vi "verify expouse time.vi"(8 "error in (no error)":errorcluster, 11 "Simulated_CCD_Camera in":refnum<class "Sim_CCD.lvclass">) -> (0 "error out":errorcluster, 3 "Simulated_CCD_Camera out":refnum<class "Sim_CCD.lvclass">)   [LabVIEW 2018, in "Sim_CCD.lvclass"]
uses:
  Sim_CCD.lvclass
  Sim_CCD.lvclass/Sim_CCD.ctl
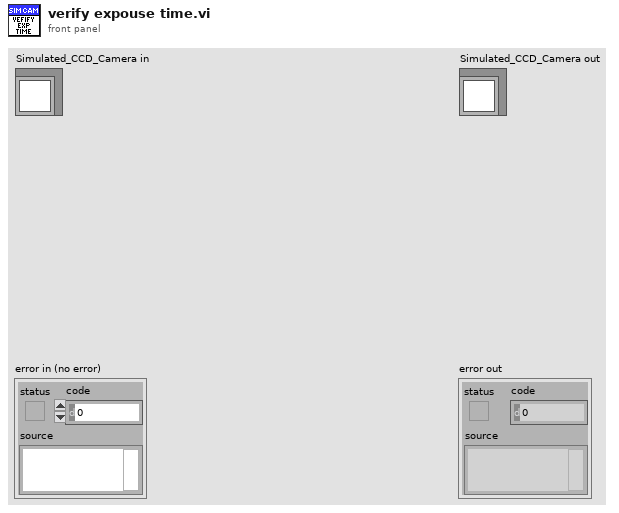
[diagram p1: front panel]
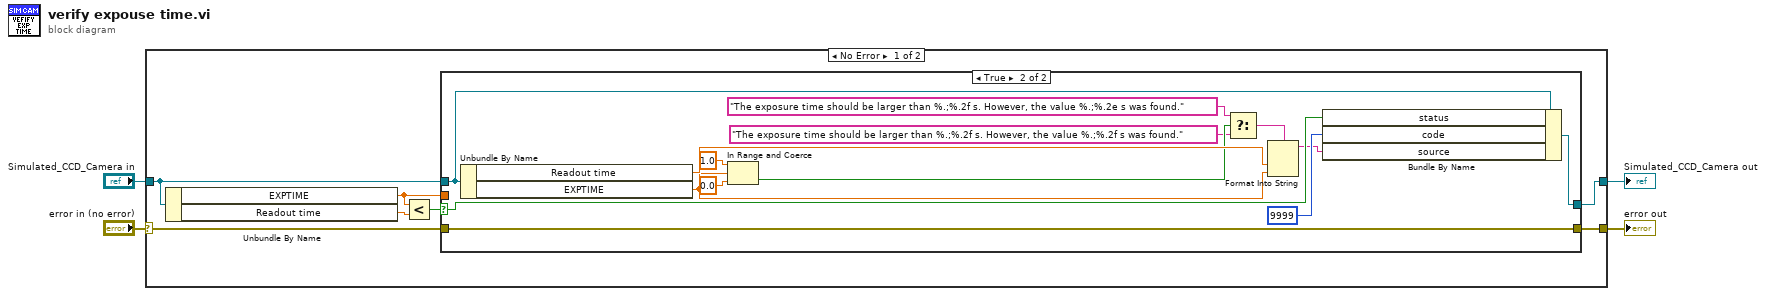
[diagram p0: block diagram]
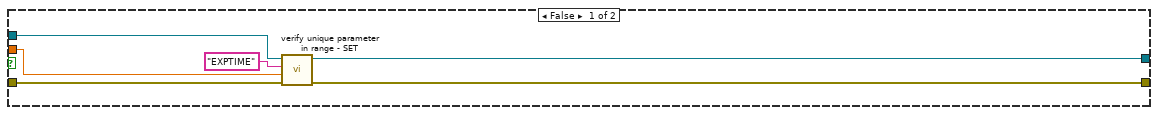
[diagram p2: hidden frame]
diagram:
  n1 = case shown="No Error" "error in (no error)" {
    selector: "error in (no error)" -> [w8 w33]
    tunnel: [w6 w33] -> w3
    tunnel: [w9 w32] -> w2
    tunnel: "Simulated_CCD_Camera in" -> [w5 w32]
    frame No Error {
      n2 = Unbundle By Name(w5) -> ("EXPTIME"=w7:dbl, "Readout time"=w11:dbl)
      n3 = Less?(x=w7, y=w11) -> (x < y?=w10:bool)
      n4 = case shown="True" w10 {
        selector: w10 -> [_ w30]
        tunnel: [w13 w31] -> w9
        tunnel: w8 -> [w17 w18]
        tunnel: w7 -> [w16 _]
        tunnel: w5 -> [w15 w19]
        tunnel: [w14 w18] -> w6
        frame False {
          n5 = call "verify unique parameter in range - SET.vi"("error in (no error)"=w17, "value"=w16, "parameter name"="EXPTIME", "Simulated_CCD_Camera in"=w15) -> ("error out"=w14:errorcluster, "Simulated_CCD_Camera out"=w13:refnum<class "Sim_CCD.lvclass">)  [unwired: 6 in]
        }
        frame True {
          n6 = Unbundle By Name(w19) -> ("Readout time"=w27:dbl, "EXPTIME"=w25:dbl)
          n7 = In Range and Coerce(upper limit=1.0, x=w25, lower limit=0.0 ("upper limit")) -> (In Range?=w24:bool)  [unwired: 1 out]
          n8 = Select(t="The exposure time should be larger than %.;%.2f s. However, the value %.;%.2e s was found." ("format string"), s=w24, f="The exposure time should be larger than %.;%.2f s. However, the value %.;%.2f s was found." ("format string")) -> (s? t:f=w21:string)
          n9 = Format Into String(format string=w21, w27, w25) -> (resulting string=w28:string)  [unwired: 2 in, 1 out]
          n10 = Bundle By Name(cluster=w19, "status"=w30, "code"=9999 ("SET errors.exposure time.code"), "source"=w28) -> (w31:refnum<class "Sim_CCD.lvclass">)
        }
      }
    }
    frame Error {
    }
  }
  "error out" <- w3
  "Simulated_CCD_Camera out" <- w2
